vi "CBindFlag.vi"(8 "error in (no error)":errorcluster, 10 "Authenticate Extra  Data":T1, 11 "WampScramAuthenticator in":refnum<class "WampScramAuthenticator.lvclass">) -> (0 "error out":errorcluster, 1 "CBindFlag":string, 2 "Authenticate Extra  Data":T1, 3 "WampScramAuthenticator out":refnum<class "WampScramAuthenticator.lvclass">)   [LabVIEW 2020, in "wamplv.lvlib" / "WampScramAuthenticator.lvclass"]
uses:
  WampScramAuthenticator.lvclass
  TypeDefs/Authenticate Extra data.ctl
  WampScramAuthenticator.lvclass/WampScramAuthenticator.ctl
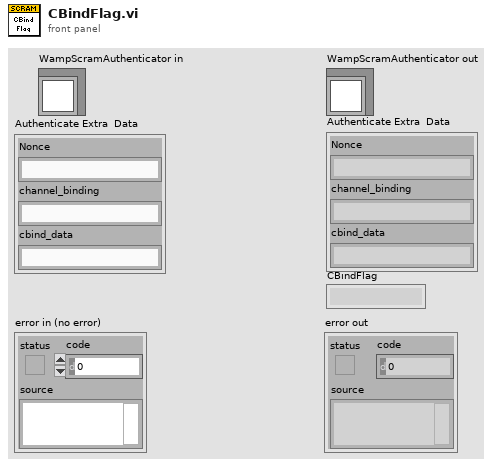
[diagram p1: front panel]
types:
  T1 = typedef "wamplv.lvlib/WampScramAuthenticator.lvclass/Authenticate Extra data.ctl" = cluster{"Nonce":string, "channel_binding":string, "cbind_data":string}
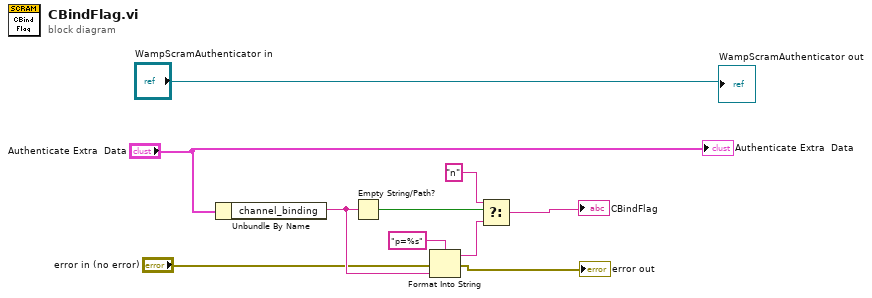
[diagram p0: block diagram]
diagram:
  n1 = Unbundle By Name("Authenticate Extra  Data") -> ("channel_binding"=w5:string)
  n2 = Empty String/Path?(string/path=w5) -> (empty?=w8:bool)
  n3 = Format Into String(format string="p=%s", error in="error in (no error)", w5) -> (resulting string=w6:string, error out=→"error out":errorcluster)  [unwired: 1 in]
  n4 = Select(t="n" ("format string"), s=w8, f=w6) -> (s? t:f=→"CBindFlag":string)
  "WampScramAuthenticator out" <- "WampScramAuthenticator in"
  "Authenticate Extra  Data" <- "Authenticate Extra  Data"
